vi "parse action report.vi"(8 "error in":errorcluster, 11 "message data":string) -> (0 "error out":errorcluster, 2 "command error":errorcluster, 3 "commands":T1)   [LabVIEW 2013, in "module execution process.lvlib"]
doc: "Returns the status of commands sent to the Engine Service that don't require additional data in the response. It will report back which command was most recently executed and if an error occurred during the execution."
uses:
  module execution process.lvlib
  command commands to rtexe process.ctl
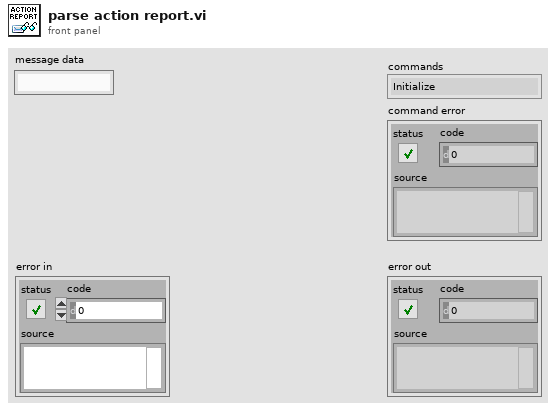
[diagram p1: front panel]
types:
  T1 = typedef "module execution process.lvlib/command commands to rtexe process.ctl" = enum16{"Initialize", "Add Search Paths", "Load from File", "Unload File", "Open All Engines", "Open Single Engine", "Initialize All Engines", "Initialize Single Engine", "Start All", "Start Single", "Pause All", "Pause Single", "Stop All", "Stop Single", "Close All", "Close Single", "Set Safe State All", "Set Safe State Single", "Get Status", "Exit", "Error", "Load Bitfile", "Unload Bitfile", "Clear Faults Single", "Clear Faults All"}
  T2 = cluster{"command string":string, "command error":errorcluster}
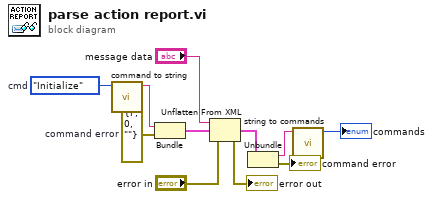
[diagram p0: block diagram]
diagram:
  w8 = errorcluster {"status"=FALSE, "code"=0, "source"=""}  # command error
  w10 = command_commands_to_rtexe_process."Initialize"  # cmd
  n1 = call "command to string.vi"("commands"=w10) -> ("command string"=w9:string)  [unwired: 10 in]
  n2 = Bundle("command string"=w9, "command error"=w8) -> (w4:T2)  [unwired: 1 in]
  n3 = Unflatten From XML(xml string="message data", type=w4, error in (no error)="error in") -> (value=w2:T2, error out=→"error out":errorcluster)
  n4 = Unbundle(w2) -> ("command string"=w7:string, "command error"=→"command error":errorcluster)
  n5 = call "string to commands.vi"("command string"=w7) -> ("commands"=→"commands":T1)  [unwired: 9 in, 1 out]
